vi "RunOperationCore.vi"(8 "error in (no error)":errorcluster, 10 "Test Report":refnum<class "Test Report.lvclass">, 11 "Project":refnum<vi>) -> (0 "error out":errorcluster)   [LabVIEW 2013, in "Test.lvclass"]
uses:
  Test.lvclass
  <vilib>/addons/_JKI Toolkits/Caraya/classes/Test Runner.Project/Test Runner.Project.lvclass
  <vilib>/addons/_JKI Toolkits/Caraya/classes/Test Runner/Test Runner.lvclass
  <vilib>/addons/_JKI Toolkits/Caraya/classes/Test Report/Test Report.lvclass
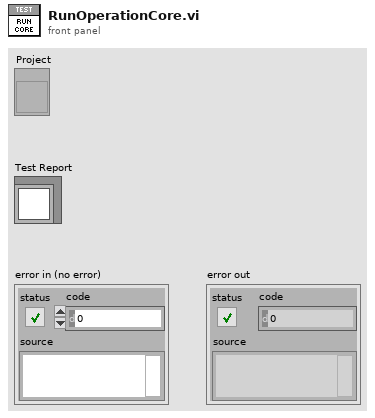
[diagram p1: front panel]
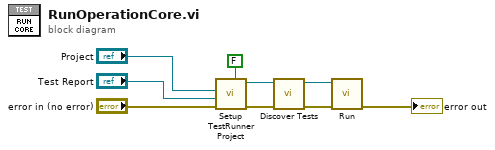
[diagram p0: block diagram]
diagram:
  n1 = call <vilib>:"Setup TestRunner Project.vi"("Interactive (T)"=FALSE, "error in (no error)"="error in (no error)", "Test Report"="Test Report", "Project Refnum"="Project") -> ("error out"=w8:errorcluster, "Test Runner.Project out"=w9:refnum<class "Test Runner.Project.lvclass">)  [unwired: 6 in]
  n2 = call <vilib>:"Discover Tests.vi"("error in (no error)"=w8, "Test Runner in"=w9) -> ("error out"=w7:errorcluster, "Test Runner out"=w6:refnum<class "Test Runner.Project.lvclass">)  [unwired: 8 in]
  n3 = call <vilib>:"Run.vi"("error in (no error)"=w7, "Test Runner in"=w6) -> ("error out"=→"error out":errorcluster)  [unwired: 7 in, 2 out]
